vi "Connect.vi"(8 "error in":errorcluster, 11 "6700C in":refnum<class "6700C.lvclass">) -> (0 "error out":errorcluster, 3 "6700C out":refnum<class "6700C.lvclass">)   [LabVIEW 2019, in "6700C.lvlib" / "6700C.lvclass"]
uses:
  Library/6700C.lvclass
  C:/Users/Public/Documents/Development/builds/Instruments/Instruments.lvlibp/Library/Instruments.lvclass
  Library/6700C.lvclass/6700C.ctl
  builds/Instruments/Instruments.lvlibp/Accessors/Read Resource.vi
  <instrlib>/Agilent N6700 Series/Agilent N6700 Series.lvlib
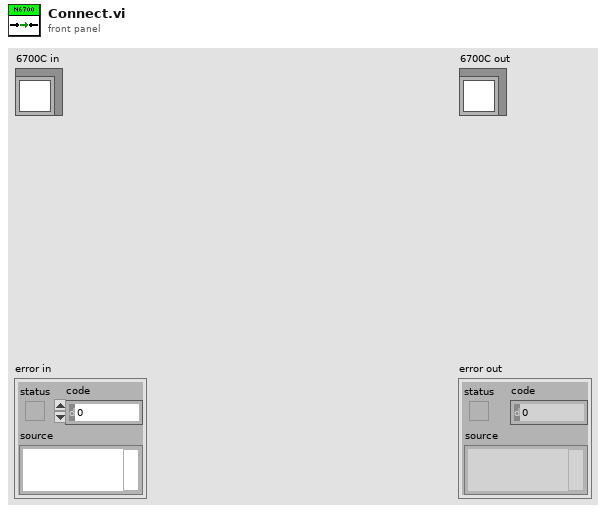
[diagram p1: front panel]
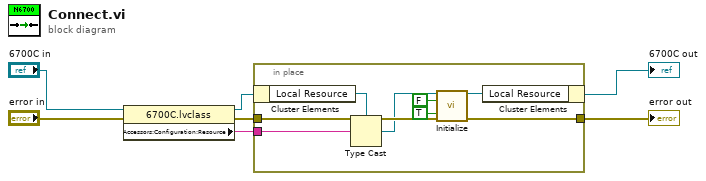
[diagram p0: block diagram]
diagram:
  n1 = property class="6700C.lvclass"(reference="6700C in", error in="error in") -> (reference out=w1:refnum<class "6700C.lvclass">, error out=w3:errorcluster, "Accessors:Configuration:Resource"=w2:string)
  n2 = in-place {
    in-place-border: w3 -> [w15]
    in-place-border: [w10] -> w4
    in-place-border: w2 -> [w14]
    n3 = in-place-cluster #1(w1) -> ("Local Resource"=w13:refnum<visa-resource-name>)
    n4 = Type Cast(type=w13, x=w14) -> (*(type *) &x=w12:refnum<visa-resource-name>)
    n5 = call <instrlib>:"Initialize.vi"("VISA resource name"=w12, "ID Query? (T: Yes)"=FALSE, "Reset? (T: Yes)"=TRUE, "error in (no error)"=w15) -> ("VISA resource name out"=w11:refnum<visa-resource-name>, "error out"=w10:errorcluster)  [unwired: 10 in]
    n6 = in-place-cluster #1("Local Resource"=w11) -> (→"6700C out":refnum<class "6700C.lvclass">)
  }
  "error out" <- w4
